vi "CheckCurrentImproperWiring.vi"(9 "Working Current":T1, 10 "Motor":T3, 11 "Group Phasors":T2[](array[typedef])) -> (1 ">min current?":bool, 3 "wiring information":string)   [LabVIEW 2017, in "McsaAnalysisLowRate.lvlib"]
uses:
  <vilib>/addons/InsightCM/Devices/Shared/Mcsa/McsaAnalysisLowRate/McsaAnalysisLowRate.lvlib
  <vilib>/addons/InsightCM/Utilities/Analysis/MCSA/controls/McsaMotor.ctl
  <vilib>/addons/InsightCM/Utilities/Analysis/MCSA/controls/McsaChannelPhasor.ctl
  <vilib>/addons/InsightCM/Utilities/Analysis/MCSA/controls/WorkingCurrent.ctl
  <vilib>/addons/InsightCM/Utilities/Analysis/MCSA/McsaAnalysisFunctions.lvlib
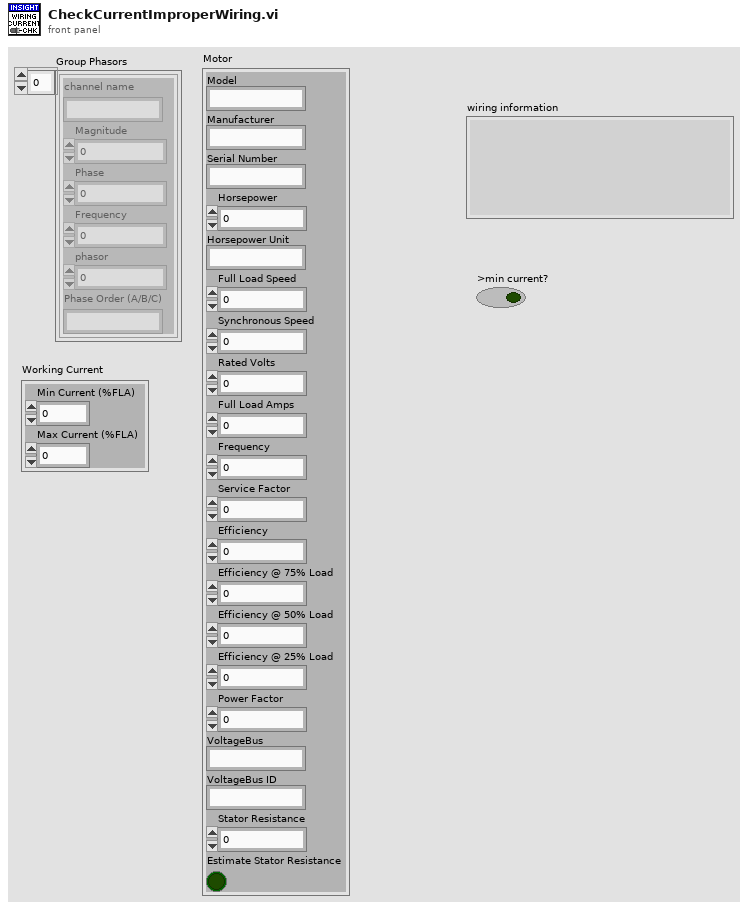
[diagram p1: front panel]
types:
  T1 = typedef "McsaAnalysisFunctions.lvlib/WorkingCurrent.ctl" = cluster{"Min Current (%FLA)":dbl, "Max Current (%FLA)":dbl}
  T2 = typedef "McsaAnalysisFunctions.lvlib/McsaChannelPhasor.ctl" = cluster{"channel name":string, "Magnitude":dbl, "Phase":dbl, "Frequency":dbl, "phasor":cdb, "Phase Order (A/B/C)":string}
  T3 = typedef "McsaAnalysisFunctions.lvlib/McsaMotor.ctl" = cluster{"Model":string, "Manufacturer":string, "Serial Number":string, "Horsepower":dbl, "Horsepower Unit":string, "Full Load Speed":dbl, "Synchronous Speed":dbl, "Rated Volts":dbl, "Full Load Amps":dbl, "Frequency":dbl, "Service Factor":dbl, "Efficiency":dbl, "Efficiency @ 75% Load":dbl, "Efficiency @ 50% Load":dbl, "Efficiency @ 25% Load":dbl, "Power Factor":dbl, "VoltageBus":string, "VoltageBus ID":string, "Stator Resistance":dbl, "Estimate Stator Resistance":bool}
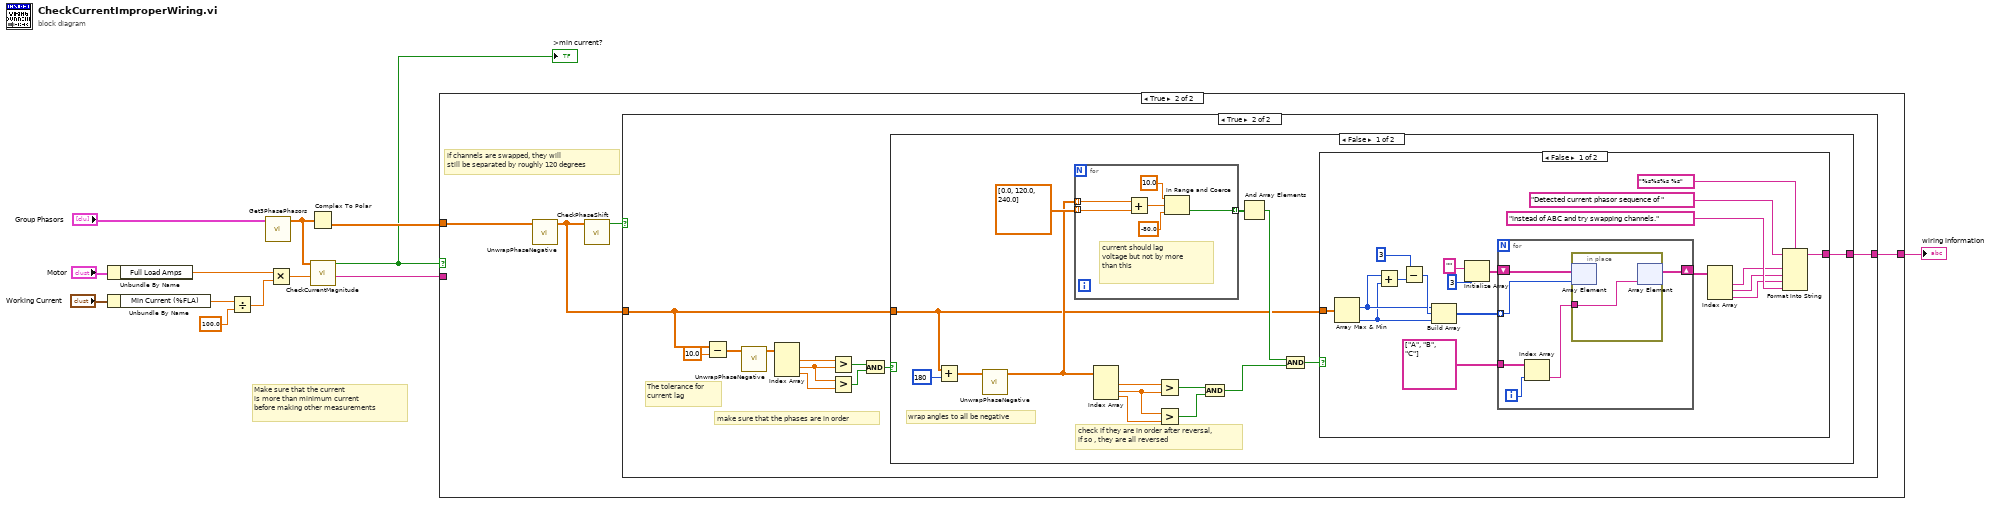
[diagram p0: block diagram]
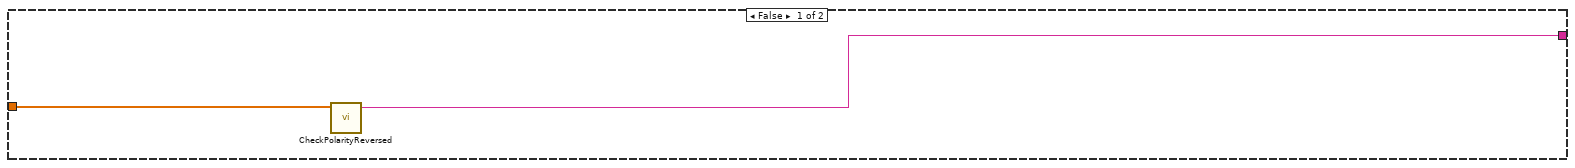
[diagram p3: hidden frame]
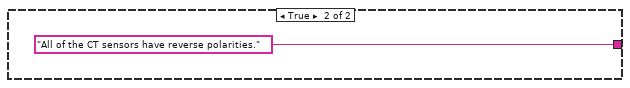
[diagram p4: hidden frame]
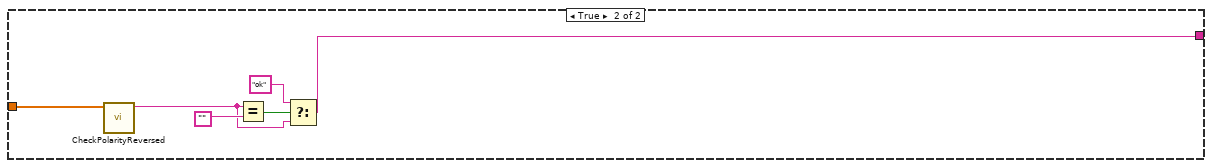
[diagram p5: hidden frame]
diagram:
  # "Make sure that the current\nis more than minimum current\nbefore making other measurements"
  n1 = Unbundle By Name("Working Current") -> ("Min Current (%FLA)"=w5:dbl)
  n2 = Unbundle By Name("Motor") -> ("Full Load Amps"=w2:dbl)
  n3 = Divide(x=w5, y=100.0) -> (x/y=w4:dbl)
  n4 = call <vilib>:"Get3PhasePhasors.vi"("Group Phasors"="Group Phasors") -> ("3-phase Phasors"=w9:cdb[])  [unwired: 10 in]
  n5 = Multiply(x=w2, y=w4) -> (x*y=w8:dbl)
  n6 = Complex To Polar(r * e^(i*theta)=w9) -> (theta=w11:dbl[])  [unwired: 1 out]
  n7 = call <vilib>:"CheckCurrentMagnitude.vi"("minimum current amps"=w8, "current phasors"=w9) -> ("wiring info"=w7:string, "> min current?"=w1:bool)  [unwired: 8 in]
  ">min current?" <- w1
  n8 = case shown="True" w1 {
    tunnel: w11 -> [_ w16]
    tunnel: [w14 w17] -> w13
    tunnel: w7 -> [w14 _]
    frame False {
    }
    frame True {
      # "if channels are swapped, they will\nstill be separated by roughly 120 degrees"
      n9 = call <vilib>:"UnwrapPhaseNegative.vi"("radian"=w16) -> ("degrees"=w15:dbl[])  [unwired: 10 in]
      n10 = call <vilib>:"CheckPhaseShift.vi"("3-phase phase degree"=w15) -> ("all 120-degree shift?"=w18:bool)  [unwired: 10 in]
      n11 = case shown="True" w18 {
        tunnel: [w19 w31] -> w17
        tunnel: w15 -> [w20 w22]
        frame False {
          n12 = call <vilib>:"CheckPolarityReversed.vi"("3-phase current phase degrees"=w20) -> ("wiring information"=w19:string)  [unwired: 10 in]
        }
        frame True {
          # "The tolerance for\ncurrent lag"
          # "make sure that the phases are in order"
          n13 = Subtract(x=w22, y=10.0 ("upper limit")) -> (x-y=w21:dbl[])
          n14 = call <vilib>:"UnwrapPhaseNegative.vi"("radian"=w21) -> ("degrees"=w23:dbl[])  [unwired: 10 in]
          n15 = Index Array(array=w23) -> (element #1=w30:dbl, element #2=w29:dbl, element #3=w28:dbl)  [unwired: 3 in]
          n16 = Greater?(x=w30, y=w29) -> (0:w26:bool)
          n17 = Greater?(x=w29, y=w28) -> (0:w27:bool)
          n18 = And(x=w26, y=w27) -> (x .and. y?=w25:bool)
          n19 = case shown="False" w25 {
            tunnel: [w46 w81] -> w31
            tunnel: w22 -> [w32 w85]
            frame False {
              # "wrap angles to all be negative"
              # "check if they are in order after reversal,\nif so , they are all reversed"
              n20 = Add(x=w32, y=180) -> (x+y=w33:dbl[])
              n21 = call <vilib>:"UnwrapPhaseNegative.vi"("radian"=w33) -> ("degrees"=w34:dbl[])  [unwired: 10 in]
              n22 = for {
                tunnel: dbl[] [0.0, 120.0, 240.0] -> [w49] mode=indexing
                tunnel: w34 -> [w48] mode=indexing
                tunnel: [w47] -> w38 mode=indexing
                # "current should lag \nvoltage but not by more than this"
                n23 = Add(x=w48, y=w49) -> (x+y=w52:dbl)
                n24 = In Range and Coerce(upper limit=10.0, x=w52, lower limit=-80.0) -> (In Range?=w47:bool)  [unwired: 1 out]
              }
              n25 = Index Array(array=w34) -> (element #1=w41:dbl, element #2=w42:dbl, element #3=w43:dbl)  [unwired: 3 in]
              n26 = Greater?(x=w41, y=w42) -> (0:w45:bool)
              n27 = Greater?(x=w42, y=w43) -> (0:w44:bool)
              n28 = And(x=w45, y=w44) -> (x .and. y?=w36:bool)
              n29 = And Array Elements(Boolean array=w38) -> (logical AND=w35:bool)
              n30 = And(x=w35, y=w36) -> (x .and. y?=w37:bool)
              n31 = case shown="False" w37 {
                tunnel: w32 -> [w71 _]
                tunnel: [w67 "All of the CT sensors have reverse polarities."] -> w46
                frame False {
                  n32 = Array Max & Min(array=w71) -> (max index (indices)=w63:i32, min index (indices)=w62:i32)  [unwired: 2 out]
                  n33 = Add(x=w63, y=w62) -> (x+y=w70:i32)
                  n34 = Subtract(x=3, y=w70) -> (x-y=w64:i32)
                  n35 = Build Array(w63, w64, w62) -> (w61:i32[])
                  n36 = Initialize Array("", 3 ("dimension size")) -> (w54:string[])
                  n37 = for {
                    tunnel: w61 -> [w74] mode=indexing
                    tunnel: string[] ["A", "B", "C"] -> [w77]
                    shift-right: [w72] -> w59
                    shift-left: w54 -> [w75]
                    i -> [w76]
                    n38 = Index Array(array=w77, index=w76) -> (element=w73:string)
                    n39 = in-place {
                      in-place-border: w73 -> [w78]
                      n40 = in-place-array #1(w75, w74) -> ()  [unwired: 1 out]
                      n41 = in-place-array #1(w78) -> (w72:string[])  [unwired: 1 out]
                    }
                  }
                  n42 = Index Array(array=w59) -> (element #1=w58:string, element #2=w57:string, element #3=w56:string)  [unwired: 3 in]
                  n43 = Format Into String(format string="%s%s%s %s", initial string="Detected current phasor sequence of ", w58, w57, w56, "instead of ABC and try swapping channels." ("input 4")) -> (resulting string=w67:string)  [unwired: 1 in, 1 out]
                }
                frame True {
                }
              }
            }
            frame True {
              n44 = call <vilib>:"CheckPolarityReversed.vi"("3-phase current phase degrees"=w85) -> ("wiring information"=w80:string)  [unwired: 10 in]
              n45 = Equal?(x=w80, y="") -> (x = y?=w83:bool)
              n46 = Select(t="ok", s=w83, f=w80) -> (s? t:f=w81:string)
            }
          }
        }
      }
    }
  }
  "wiring information" <- w13
